vi "Forward Command.vi"(8 "error in (no error)":errorcluster, 10 "command":T1, 11 "Dispatcher in":refnum<class "Dispatcher.lvclass">) -> (0 "error out":errorcluster, 3 "Dispatcher out":refnum<class "Dispatcher.lvclass">)   [LabVIEW 2017, in "DSF Core.lvlib" / "Dispatcher.lvclass"]
uses:
  Dispatcher.lvclass
  Interfaces/Dispatcher/Command Data.ctl
  Interfaces/Dispatcher/Command.ctl
  Interfaces/Dispatcher/Parameters.ctl
  Dispatcher.lvclass/Dispatcher.ctl
  Interfaces/Dispatcher/Dispatcher Interface.lvclass
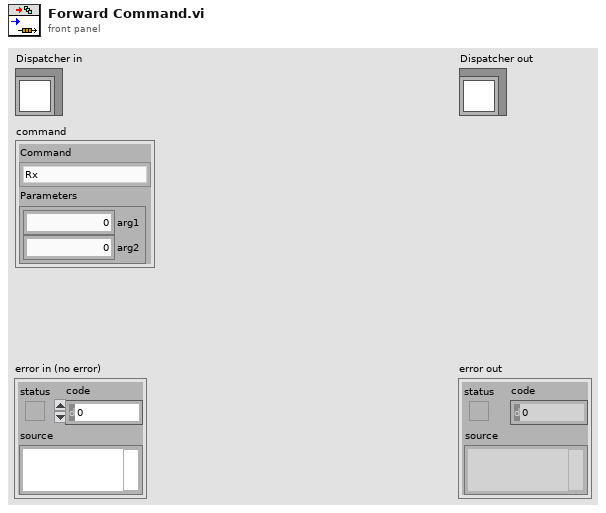
[diagram p1: front panel]
types:
  T1 = typedef "DSF Core.lvlib/Dispatcher Interface.lvclass/Command Data.ctl" = cluster{"Command":T2, "Parameters":T3}
  T2 = typedef "DSF Core.lvlib/Dispatcher Interface.lvclass/Command.ctl" = enum8{"Rx", "Tx", "Shutdown"}
  T3 = typedef "DSF Core.lvlib/Dispatcher Interface.lvclass/Parameters.ctl" = cluster{"arg1":u64, "arg2":u64}
  T4 = typedef "DSF Core.lvlib/Dispatcher Interface.lvclass/Response Data.ctl" = cluster{"Response":T5, "Parameters":T3}
  T5 = typedef "DSF Core.lvlib/Dispatcher Interface.lvclass/Response.ctl" = enum8{"General Ack", "Error", "Shutting Down"}
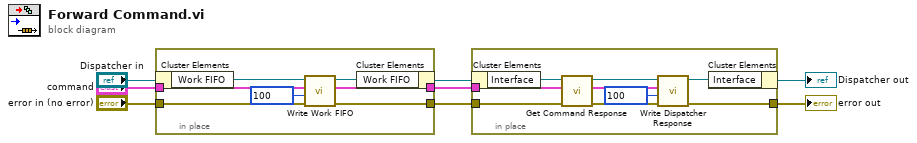
[diagram p0: block diagram]
diagram:
  n1 = in-place {
    in-place-border: "command" -> [w13]
    in-place-border: "error in (no error)" -> [w12]
    in-place-border: [w11] -> w3
    in-place-border: [w10] -> w4
    n2 = in-place-cluster #1("Dispatcher in") -> ("Work FIFO"=w15:refnum<k33>)
    n3 = call "Write Work FIFO.vi"("error in (no error)"=w12, "timeout in ms (0)"=100, "command in"=w13, "Work FIFO in"=w15) -> ("error out"=w11:errorcluster, "command out"=w10:T1, "Work FIFO out"=w14:refnum<k33>)  [unwired: 3 in, 2 out]
    n4 = in-place-cluster #1("Work FIFO"=w14) -> (w5:refnum<class "Dispatcher.lvclass">)
  }
  n5 = in-place {
    in-place-border: w4 -> [w18]
    in-place-border: w3 -> [w20]
    in-place-border: [w19] -> w1
    n6 = in-place-cluster #2(w5) -> ("Interface"=w17:refnum<class "Dispatcher Interface.lvclass">)
    n7 = call "Get Command Response.vi"("error in (no error)"=w20, "command"=w18, "Dispatcher Interface in"=w17) -> ("error out"=w23:errorcluster, "response"=w22:T4, "Dispatcher Interface out"=w24:refnum<class "Dispatcher Interface.lvclass">)  [unwired: 6 in]
    n8 = call "Write Dispatcher Response.vi"("error in (no error)"=w23, "timeout in ms (0)"=100, "response"=w22, "Dispatcher Interface in"=w24) -> ("error out"=w19:errorcluster, "Dispatcher Interface out"=w16:refnum<class "Dispatcher Interface.lvclass">)  [unwired: 5 in, 1 out]
    n9 = in-place-cluster #2("Interface"=w16) -> (→"Dispatcher out":refnum<class "Dispatcher.lvclass">)
  }
  "error out" <- w1
